vi "Main.vi"(8 "error in":errorcluster, 9 "Error Queue":refnum<queue>, 10 "Controller Queue":refnum<queue>, 11 "Application Events":refnum<user-event>) -> (0 "error out":errorcluster)   [LabVIEW 2020, in "Controller.lvlib"]
doc: "Main Vi for controller module"
uses:
  Controller.lvlib
  Controls/Module Message.ctl
  Controls/Application Modules.ctl
  Controls/Application Event Message.ctl
  Controls/Application Events.ctl
  Controls/Module Consummer Loop Data.ctl
  Controls/Module State.ctl
  Configuration Database/Configuration Database.lvlib
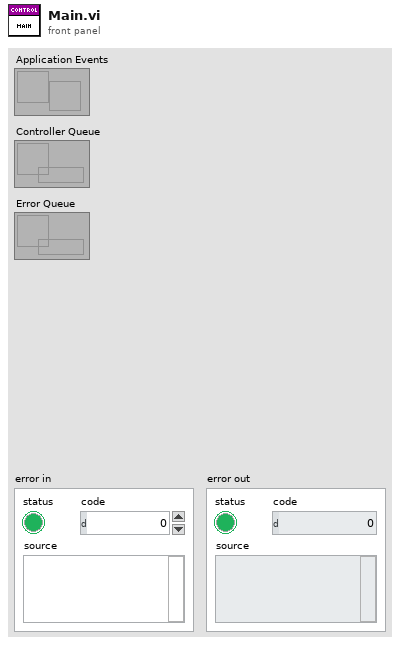
[diagram p1: front panel]
types:
  T1 = typedef "Controller.lvlib/Module State.ctl" = enum16{"Initial State", "Start And Move State", "Analysis State", "Continue Travel State", "Stop At Floor", "Open And Close Door Sequence State", "No Request Remaining State", "Emergency Call State", "Terminate Process State"}
  T2 = typedef "Controller.lvlib/Application Event Message.ctl" = cluster{"Source":T3, "Event":T4, "Data":variant}
  T3 = typedef "Controller.lvlib/Application Modules.ctl" = enum16{"Controller", "User Console", "Display Console", "Sensor Interface", "Configuration Database", "Error Module"}
  T4 = typedef "Controller.lvlib/Application Events.ctl" = enum16{"Controller: Initialize", "Controller: Initialize Start And Move State", "Controller: Initialize Analysis State", "Controller: Initialize Continue Travel State", "Controller: Initialize Stop At Floor", "Controller: Initialize Open And Close Door Sequence", "Controller: Initialize No Request Remaining", "Controller: Initialize Emergency Call", "Controller: Initialize Terminate Process", "Controller: Publish State", "UI: Elevator Call", "UI: Broadcast State", "UI: Next Destination Reached", "UI: Timeout Reached", "UI: Emergency Call", "UI: Terminate State", "UI: Door Opened", "UI: Door Closed", "UI: Floor Reached", "UI: Door About To Close"}
  T5 = typedef "Controller.lvlib/Module Consummer Loop Data.ctl" = cluster{"State Machine":cluster{"Module State":T1, "State Data":variant, "Current Operation":cluster{"Initial Floor":i32, "Elevator Calls":i32[], "Current Movement":bool}[]}}
  T6 = cluster{"Initial Floor":i32, "Elevator Calls":i32[], "Current Movement":bool}[]
  T7 = cluster{"Initial Floor":i32, "Elevator Calls":i32[], "Current Movement":bool}
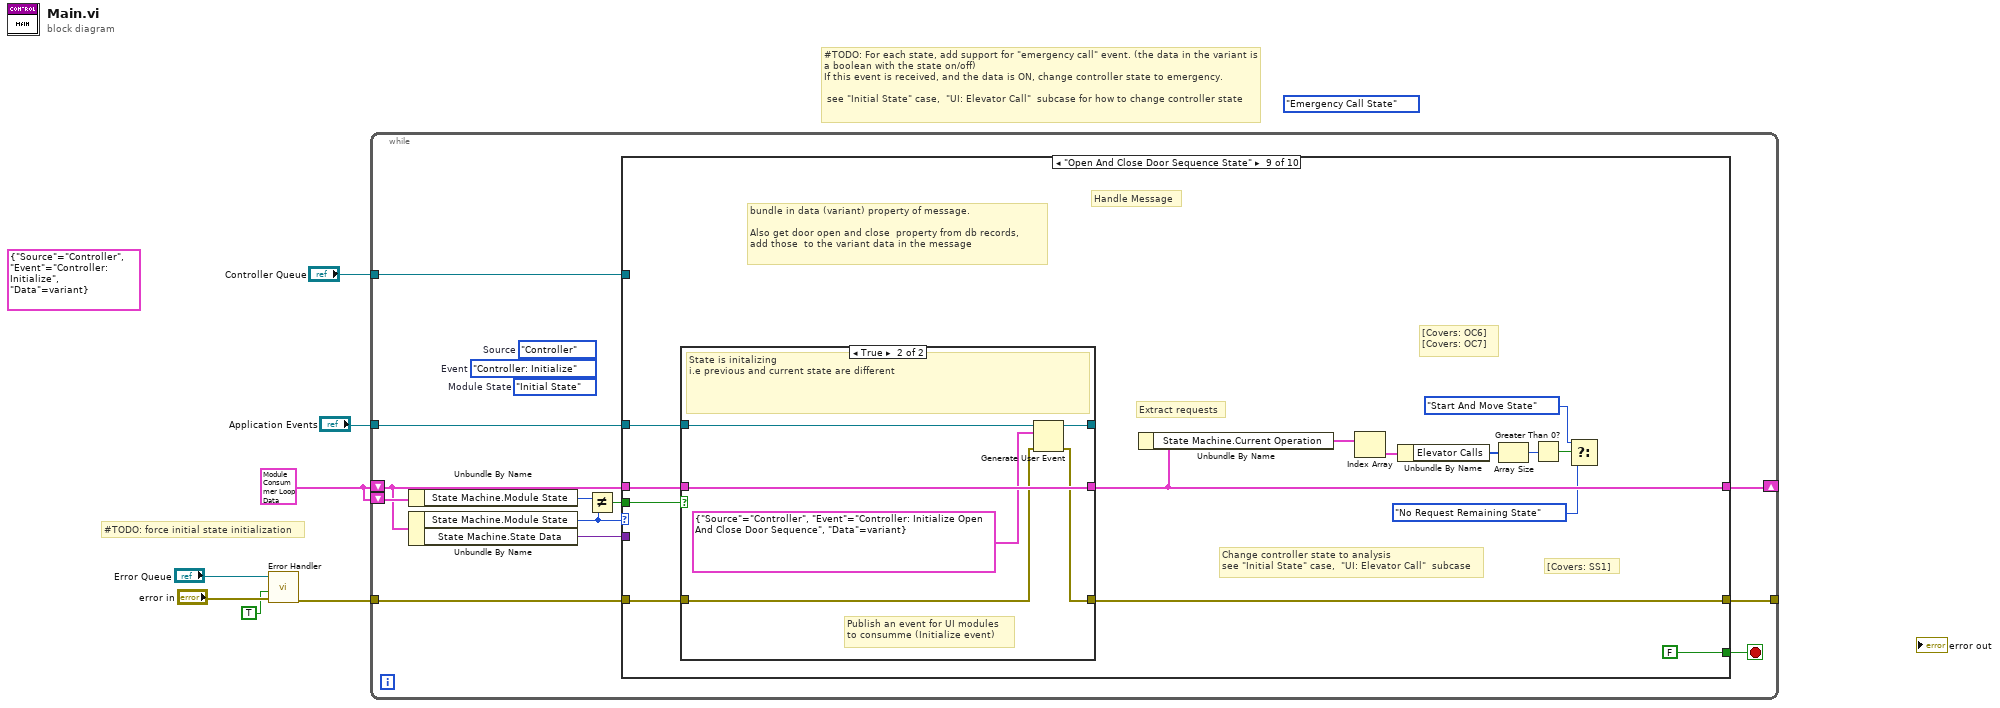
[diagram p0: block diagram]
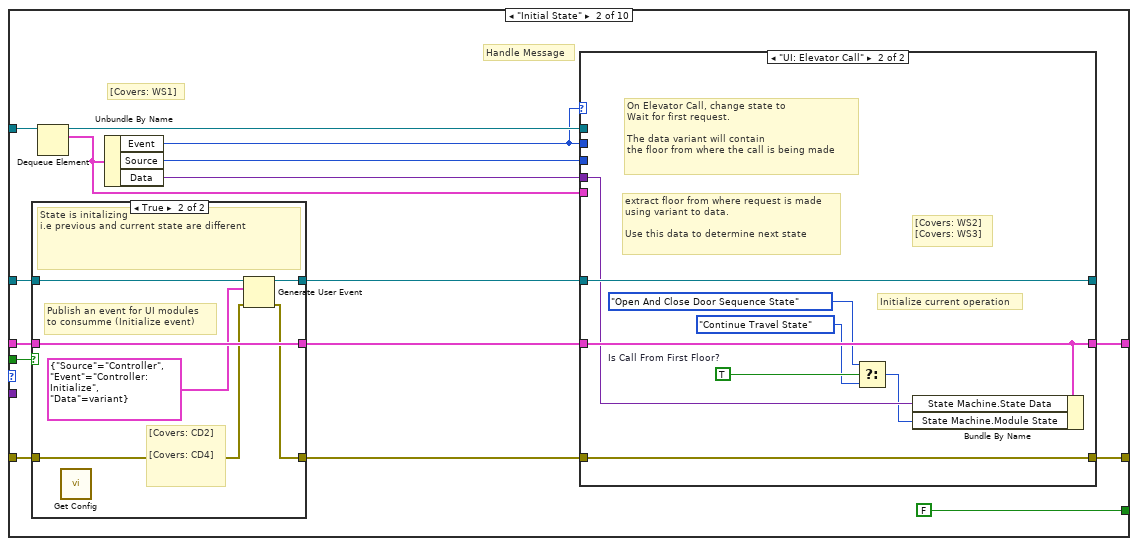
[diagram p3: hidden frame]
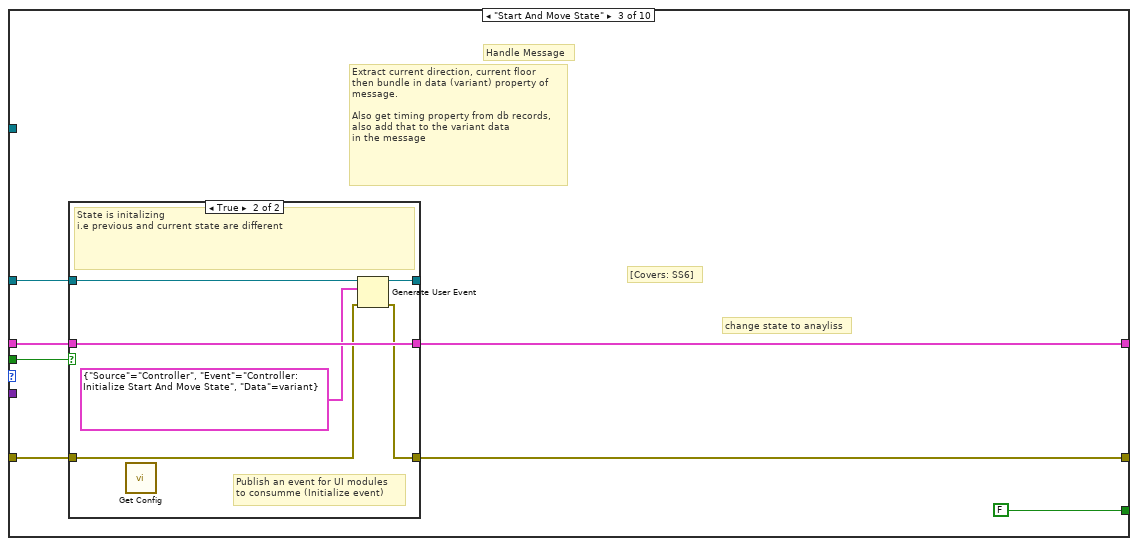
[diagram p6: hidden frame]
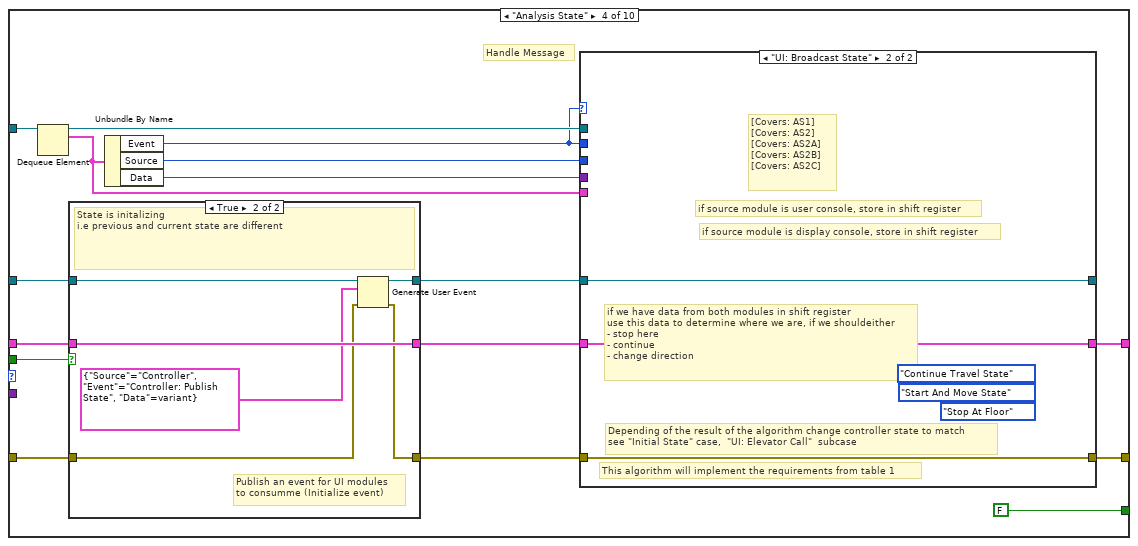
[diagram p8: hidden frame]
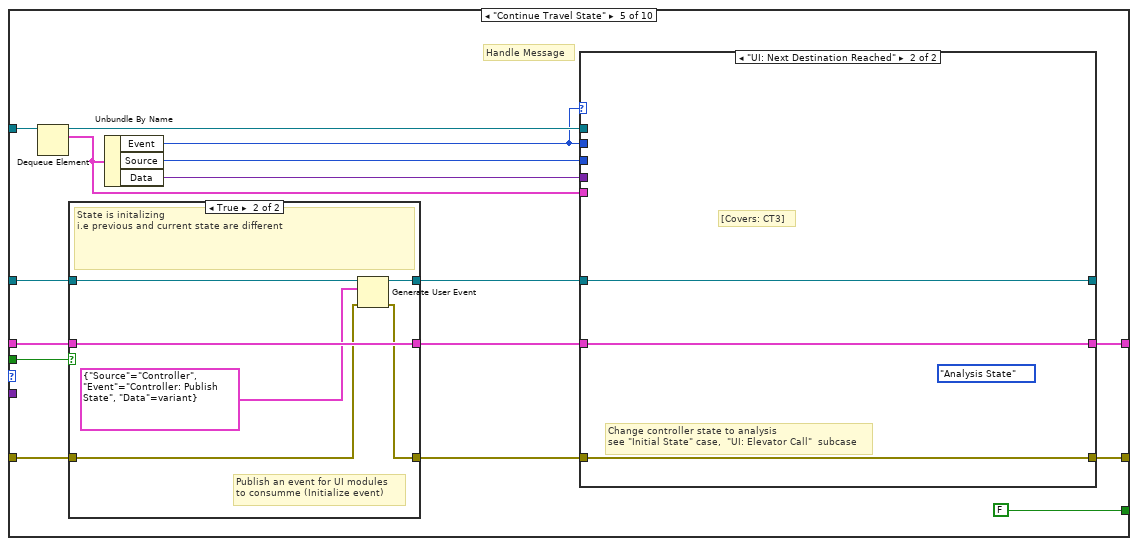
[diagram p11: hidden frame]
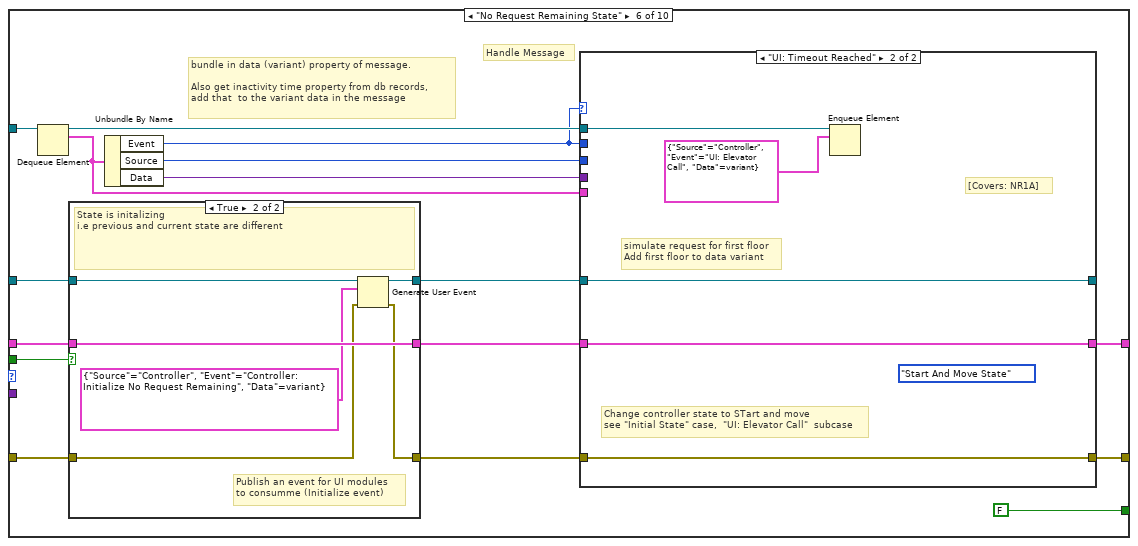
[diagram p14: hidden frame]
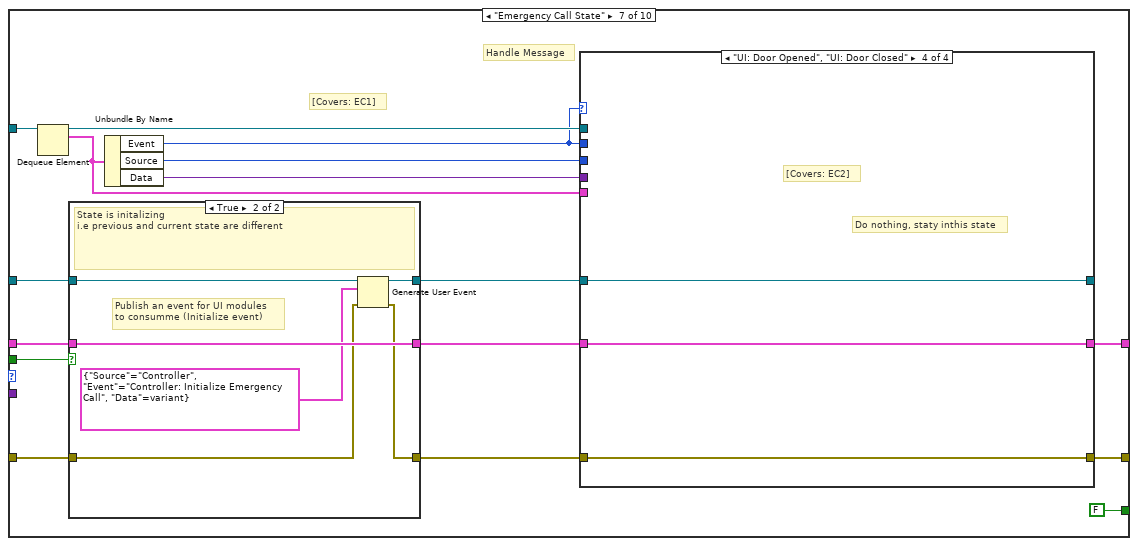
[diagram p17: hidden frame]
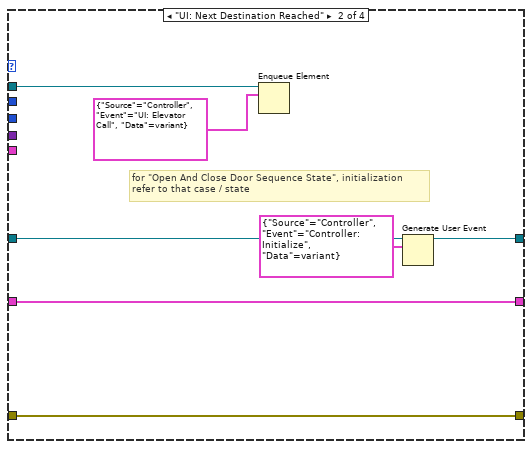
[diagram p19: hidden frame]
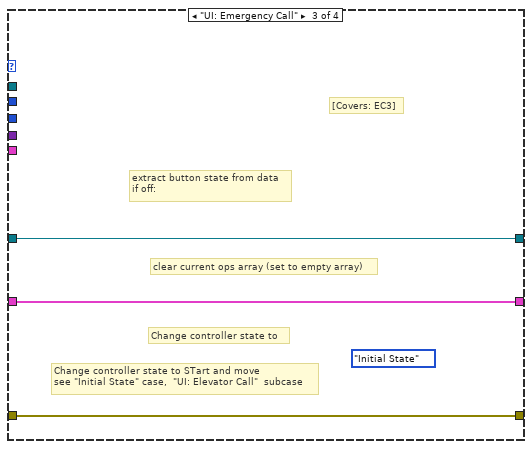
[diagram p20: hidden frame]
diagram:
  (unwired) Module_State."Emergency Call State" ("State Machine.Module State")
  (unwired) T2 {"Source"=enum."Controller", "Event"=enum."Controller: Initialize", "Data"=variant} ("Elevator Events")
  w1 = T5 {"State Machine"={"Module State"=enum."Initial State", "State Data"=variant, "Current Operation"=[]}} ("Loop Data")
  # "#TODO: For each state, add support for \"emergency call\" event. (the data in the variant is a boolean with the state on/off)\nIf this event is received, and the data is ON, change controller state to emergency.\n\n see \"Initial State\" case,  \"UI: Elevator Call\"  subcase for how to change controller state"
  # "#TODO: force initial state initialization"
  n1 = call "Error Handler.vi"("error in"="error in", "Load Reference?"=TRUE, "Error Queue"="Error Queue") -> ("error out"=w4:errorcluster)  [unwired: 8 in]
  n2 = while {
    tunnel: w4 -> [w10]
    shift-right: [w19] -> _
    shift-left: w1 -> [w17]
    shift-left: w1 -> [w18]
    tunnel: "Application Events" -> [w12]
    tunnel: "Controller Queue" -> [w11]
    tunnel: [w9] -> _
    stop <- w8 stop-if-true
    (unwired) Module_State."Initial State"  # Module State
    (unwired) Application_Events."Controller: Initialize"  # Event
    (unwired) Application_Modules."Controller"  # Source
    n3 = Unbundle By Name(w18) -> ("State Machine.Module State"=w16:T1)
    n4 = Unbundle By Name(w17) -> ("State Machine.Module State"=w15:T1, "State Machine.State Data"=w13:variant)
    n5 = Not Equal?(x=w16, y=w15) -> (x != y?=w14:bool)
    n6 = case shown="\"Open And Close Door Sequence State\"" w15 {
      tunnel: w17 -> [w21 w31 w60 w82 w112 w142 w174 w214 w239 w256]
      tunnel: [w21 w29 w58 w80 w110 w140 w172 w212 w239 w256] -> w19
      tunnel: w14 -> [_ w36 w63 w87 w117 w147 w179 w219 w244 w259]
      tunnel: w13 -> [_ _ _ _ _ _ _ _ _ _]
      tunnel: w12 -> [_ w35 w62 w86 w116 w146 w178 w218 w243 w258]
      tunnel: w11 -> [_ w34 _ w85 w115 w145 w177 w217 _ _]
      tunnel: w10 -> [w20 w33 w61 w84 w114 w144 w176 w216 w242 w257]
      tunnel: [w20 w28 w57 w79 w109 w139 w171 w211 w241 w255] -> w9
      tunnel: [_ FALSE FALSE FALSE FALSE FALSE FALSE FALSE FALSE FALSE] -> w8
      frame Default {
      }
      frame "Initial State" {
        # "[Covers: WS1]"
        # "Handle Message"
        n7 = case shown="True" w36 {
          tunnel: w31 -> [w49 w56]
          tunnel: [w49 w56] -> _
          tunnel: w35 -> [w48 w55]
          tunnel: w33 -> [w50 w52]
          tunnel: [w50 w51] -> w30
          tunnel: [w48 w54] -> w32
          frame False {
          }
          frame True {
            # "[Covers: CD2] \n\n[Covers: CD4]"
            # "Publish an event for UI modules\nto consumme (Initialize event)"
            # "State is initalizing\ni.e previous and current state are different"
            n8 = call "Get Config.vi"() -> ()  [unwired: 11 in, 1 out]
            n9 = Generate User Event(user event=w55, event data cluster=T2 {"Source"=enum."Controller", "Event"=enum."Controller: Initialize", "Data"=variant} ("event data"), error in=w52) -> (user event out=w54:refnum<user-event>, error out=w51:errorcluster)  [unwired: 1 in]
          }
        }
        n10 = Dequeue Element(queue=w34) -> (queue out=w27:refnum<queue>, element=w26:T2)  [unwired: 2 in, 2 out]
        n11 = Unbundle By Name(w26) -> ("Event"=w22:T4, "Source"=w24:T3, "Data"=w25:variant)
        n12 = case shown="\"UI: Elevator Call\"" w22 {
          tunnel: w31 -> [w38 w45]
          tunnel: [w38 w45] -> w29
          tunnel: w32 -> [w37 w46]
          tunnel: w30 -> [w39 w47]
          tunnel: [w39 w47] -> w28
          tunnel: [w37 w46] -> _
          tunnel: w27 -> [_ _]
          tunnel: w26 -> [_ _]
          tunnel: w25 -> [_ w44]
          tunnel: w24 -> [_ _]
          tunnel: w22 -> [_ _]
          frame Default {
          }
          frame "UI: Elevator Call" {
            w43 = TRUE  # Is Call From First Floor?
            # "Initialize current operation"
            # "[Covers: WS2] \n[Covers: WS3]"
            # "extract floor from where request is made\nusing variant to data.\n\nUse this data to determine next state"
            # "On Elevator Call, change state to\nWait for first request.\n\nThe data variant will contain\nthe floor from where the call is being made"
            n13 = Select(t=Module_State."Open And Close Door Sequence State" ("State Machine.Module State"), s=w43, f=Module_State."Continue Travel State" ("State Machine.Module State")) -> (s? t:f=w42:T1)
            n14 = Bundle By Name(cluster=w45, "State Machine.State Data"=w44, "State Machine.Module State"=w42) -> ()  [unwired: 1 out]
          }
        }
      }
      frame "Start And Move State" {
        # "change state to anayliss"
        # "[Covers: SS6]"
        # "Extract current direction, current floor\nthen bundle in data (variant) property of message.\n\nAlso get timing property from db records, also add that to the variant data\nin the message"
        # "Handle Message"
        n15 = case shown="True" w63 {
          tunnel: w60 -> [w65 w72]
          tunnel: [w65 w72] -> w58
          tunnel: w62 -> [w64 w71]
          tunnel: w61 -> [w66 w68]
          tunnel: [w66 w67] -> w57
          tunnel: [w64 w70] -> _
          frame False {
          }
          frame True {
            # "Publish an event for UI modules\nto consumme (Initialize event)"
            # "State is initalizing\ni.e previous and current state are different"
            n16 = call "Get Config.vi"() -> ()  [unwired: 11 in, 1 out]
            n17 = Generate User Event(user event=w71, event data cluster=T2 {"Source"=enum."Controller", "Event"=enum."Controller: Initialize Start And Move State", "Data"=variant} ("event data"), error in=w68) -> (user event out=w70:refnum<user-event>, error out=w67:errorcluster)  [unwired: 1 in]
          }
        }
      }
      frame "Analysis State" {
        # "Handle Message"
        n18 = Dequeue Element(queue=w85) -> (queue out=w78:refnum<queue>, element=w77:T2)  [unwired: 2 in, 2 out]
        n19 = case shown="True" w87 {
          tunnel: w82 -> [w95 w102]
          tunnel: [w95 w102] -> _
          tunnel: w86 -> [w94 w101]
          tunnel: w84 -> [w96 w98]
          tunnel: [w96 w97] -> w81
          tunnel: [w94 w100] -> w83
          frame False {
          }
          frame True {
            # "Publish an event for UI modules\nto consumme (Initialize event)"
            # "State is initalizing\ni.e previous and current state are different"
            n20 = Generate User Event(user event=w101, event data cluster=T2 {"Source"=enum."Controller", "Event"=enum."Controller: Publish State", "Data"=variant} ("event data"), error in=w98) -> (user event out=w100:refnum<user-event>, error out=w97:errorcluster)  [unwired: 1 in]
          }
        }
        n21 = Unbundle By Name(w77) -> ("Event"=w73:T4, "Source"=w75:T3, "Data"=w76:variant)
        n22 = case shown="\"UI: Broadcast State\"" w73 {
          tunnel: w82 -> [w89 w93]
          tunnel: [w89 w93] -> w80
          tunnel: w83 -> [w88 w91]
          tunnel: w81 -> [w90 w92]
          tunnel: [w90 w92] -> w79
          tunnel: [w88 w91] -> _
          tunnel: w78 -> [_ _]
          tunnel: w77 -> [_ _]
          tunnel: w76 -> [_ _]
          tunnel: w75 -> [_ _]
          tunnel: w73 -> [_ _]
          frame Default {
          }
          frame "UI: Broadcast State" {
            (unwired) Module_State."Stop At Floor" ("State Machine.Module State")
            (unwired) Module_State."Start And Move State" ("State Machine.Module State")
            (unwired) Module_State."Continue Travel State" ("State Machine.Module State")
            # "[Covers: AS1] \n[Covers: AS2] \n[Covers: AS2A] \n[Covers: AS2B] \n[Covers: AS2C]"
            # "Depending of the result of the algorithm change controller state to match\nsee \"Initial State\" case,  \"UI: Elevator Call\"  subcase"
            # "This algorithm will implement the requirements from table 1"
            # "if we have data from both modules in shift register\nuse this data to determine where we are, if we shouldeither\n- stop here\n- continue\n- change direction"
            # "if source module is display console, store in shift register"
            # "if source module is user console, store in shift register"
          }
        }
      }
      frame "Continue Travel State" {
        # "Handle Message"
        n23 = Dequeue Element(queue=w115) -> (queue out=w108:refnum<queue>, element=w107:T2)  [unwired: 2 in, 2 out]
        n24 = case shown="True" w117 {
          tunnel: w112 -> [w125 w132]
          tunnel: [w125 w132] -> _
          tunnel: w116 -> [w124 w131]
          tunnel: w114 -> [w126 w128]
          tunnel: [w126 w127] -> w111
          tunnel: [w124 w130] -> w113
          frame False {
          }
          frame True {
            # "Publish an event for UI modules\nto consumme (Initialize event)"
            # "State is initalizing\ni.e previous and current state are different"
            n25 = Generate User Event(user event=w131, event data cluster=T2 {"Source"=enum."Controller", "Event"=enum."Controller: Publish State", "Data"=variant} ("event data"), error in=w128) -> (user event out=w130:refnum<user-event>, error out=w127:errorcluster)  [unwired: 1 in]
          }
        }
        n26 = Unbundle By Name(w107) -> ("Event"=w103:T4, "Source"=w105:T3, "Data"=w106:variant)
        n27 = case shown="\"UI: Next Destination Reached\"" w103 {
          tunnel: w112 -> [w119 w123]
          tunnel: [w119 w123] -> w110
          tunnel: w113 -> [w118 w121]
          tunnel: w111 -> [w120 w122]
          tunnel: [w120 w122] -> w109
          tunnel: [w118 w121] -> _
          tunnel: w108 -> [_ _]
          tunnel: w107 -> [_ _]
          tunnel: w106 -> [_ _]
          tunnel: w105 -> [_ _]
          tunnel: w103 -> [_ _]
          frame Default {
          }
          frame "UI: Next Destination Reached" {
            (unwired) Module_State."Analysis State" ("State Machine.Module State")
            # "[Covers: CT3]"
            # "Change controller state to analysis\nsee \"Initial State\" case,  \"UI: Elevator Call\"  subcase"
          }
        }
      }
      frame "No Request Remaining State" {
        # "bundle in data (variant) property of message.\n\nAlso get inactivity time property from db records, \nadd that  to the variant data in the message"
        # "Handle Message"
        n28 = Dequeue Element(queue=w145) -> (queue out=w138:refnum<queue>, element=w137:T2)  [unwired: 2 in, 2 out]
        n29 = case shown="True" w147 {
          tunnel: w142 -> [w157 w164]
          tunnel: [w157 w164] -> _
          tunnel: w146 -> [w156 w163]
          tunnel: w144 -> [w158 w160]
          tunnel: [w158 w159] -> w141
          tunnel: [w156 w162] -> w143
          frame False {
          }
          frame True {
            # "Publish an event for UI modules\nto consumme (Initialize event)"
            # "State is initalizing\ni.e previous and current state are different"
            n30 = Generate User Event(user event=w163, event data cluster=T2 {"Source"=enum."Controller", "Event"=enum."Controller: Initialize No Request Remaining", "Data"=variant} ("event data"), error in=w160) -> (user event out=w162:refnum<user-event>, error out=w159:errorcluster)  [unwired: 1 in]
          }
        }
        n31 = Unbundle By Name(w137) -> ("Event"=w133:T4, "Source"=w135:T3, "Data"=w136:variant)
        n32 = case shown="\"UI: Timeout Reached\"" w133 {
          tunnel: w142 -> [w149 w155]
          tunnel: [w149 w155] -> w140
          tunnel: w143 -> [w148 w153]
          tunnel: w141 -> [w150 w154]
          tunnel: [w150 w154] -> w139
          tunnel: [w148 w153] -> _
          tunnel: w138 -> [_ w152]
          tunnel: w137 -> [_ _]
          tunnel: w136 -> [_ _]
          tunnel: w135 -> [_ _]
          tunnel: w133 -> [_ _]
          frame Default {
          }
          frame "UI: Timeout Reached" {
            (unwired) Module_State."Start And Move State" ("State Machine.Module State")
            # "[Covers: NR1A]"
            # "simulate request for first floor\nAdd first floor to data variant"
            # "Change controller state to STart and move\nsee \"Initial State\" case,  \"UI: Elevator Call\"  subcase"
            n33 = Enqueue Element(queue=w152, element=T2 {"Source"=enum."Controller", "Event"=enum."UI: Elevator Call", "Data"=variant}) -> ()  [unwired: 2 in, 3 out]
          }
        }
      }
      frame "Emergency Call State" {
        # "[Covers: EC1]"
        # "Handle Message"
        n34 = Dequeue Element(queue=w177) -> (queue out=w170:refnum<queue>, element=w169:T2)  [unwired: 2 in, 2 out]
        n35 = case shown="True" w179 {
          tunnel: w174 -> [w197 w204]
          tunnel: [w197 w204] -> _
          tunnel: w178 -> [w196 w203]
          tunnel: w176 -> [w198 w200]
          tunnel: [w198 w199] -> w173
          tunnel: [w196 w202] -> w175
          frame False {
          }
          frame True {
            # "Publish an event for UI modules\nto consumme (Initialize event)"
            # "State is initalizing\ni.e previous and current state are different"
            n36 = Generate User Event(user event=w203, event data cluster=T2 {"Source"=enum."Controller", "Event"=enum."Controller: Initialize Emergency Call", "Data"=variant} ("event data"), error in=w200) -> (user event out=w202:refnum<user-event>, error out=w199:errorcluster)  [unwired: 1 in]
          }
        }
        n37 = Unbundle By Name(w169) -> ("Event"=w165:T4, "Source"=w167:T3, "Data"=w168:variant)
        n38 = case shown="\"UI: Door Opened\", \"UI: Door Closed\"" w165 {
          tunnel: w174 -> [w181 w189 w192 w195]
          tunnel: [w181 w189 w192 w195] -> w172
          tunnel: w175 -> [w180 w185 w190 w193]
          tunnel: w173 -> [w182 w188 w191 w194]
          tunnel: [w182 w188 w191 w194] -> w171
          tunnel: [w180 w184 w190 w193] -> _
          tunnel: w170 -> [_ w187 _ _]
          tunnel: w169 -> [_ _ _ _]
          tunnel: w168 -> [_ _ _ _]
          tunnel: w167 -> [_ _ _ _]
          tunnel: w165 -> [_ _ _ _]
          frame Default {
          }
          frame "UI: Next Destination Reached" {
            # "for \"Open And Close Door Sequence State\", initialization\nrefer to that case / state"
            n39 = Enqueue Element(queue=w187, element=T2 {"Source"=enum."Controller", "Event"=enum."UI: Elevator Call", "Data"=variant}) -> ()  [unwired: 2 in, 3 out]
            n40 = Generate User Event(user event=w185, event data cluster=T2 {"Source"=enum."Controller", "Event"=enum."Controller: Initialize", "Data"=variant} ("event data")) -> (user event out=w184:refnum<user-event>)  [unwired: 2 in, 1 out]
          }
          frame "UI: Emergency Call" {
            (unwired) Module_State."Initial State" ("State Machine.Module State")
            # "[Covers: EC3]"
            # "Change controller state to STart and move\nsee \"Initial State\" case,  \"UI: Elevator Call\"  subcase"
            # "Change controller state to"
            # "clear current ops array (set to empty array)"
            # "extract button state from data\nif off:"
          }
          frame "UI: Door Opened", "UI: Door Closed" {
            # "Do nothing, staty inthis state"
            # "[Covers: EC2]"
          }
        }
      }
      frame "Terminate Process State" {
        # "Handle Message"
        n41 = Dequeue Element(queue=w217) -> (queue out=w210:refnum<queue>, element=w209:T2)  [unwired: 2 in, 2 out]
        n42 = case shown="True" w219 {
          tunnel: w214 -> [w224 w231]
          tunnel: [w224 w231] -> _
          tunnel: w218 -> [w223 w230]
          tunnel: w216 -> [w225 w227]
          tunnel: [w225 w226] -> w213
          tunnel: [w223 w229] -> w215
          frame False {
          }
          frame True {
            # "Publish an event for UI modules\nto consumme (Initialize event)"
            # "State is initalizing\ni.e previous and current state are different"
            n43 = Generate User Event(user event=w230, event data cluster=T2 {"Source"=enum."Controller", "Event"=enum."Controller: Initialize Terminate Process", "Data"=variant} ("event data"), error in=w227) -> (user event out=w229:refnum<user-event>, error out=w226:errorcluster)  [unwired: 1 in]
          }
        }
        n44 = Unbundle By Name(w209) -> ("Event"=w205:T4, "Source"=w207:T3, "Data"=w208:variant)
        n45 = case shown="Default" w205 {
          tunnel: w214 -> [w221]
          tunnel: [w221] -> w212
          tunnel: w215 -> [w220]
          tunnel: w213 -> [w222]
          tunnel: [w222] -> w211
          tunnel: [w220] -> _
          tunnel: w210 -> [_]
          tunnel: w209 -> [_]
          tunnel: w208 -> [_]
          tunnel: w207 -> [_]
          tunnel: w205 -> [_]
          frame Default {
          }
        }
      }
      frame "Open And Close Door Sequence State" {
        # "[Covers: SS1]"
        # "[Covers: OC6]\n[Covers: OC7]"
        # "Extract requests"
        # "Change controller state to analysis\nsee \"Initial State\" case,  \"UI: Elevator Call\"  subcase"
        # "bundle in data (variant) property of message.\n\nAlso get door open and close  property from db records, \nadd those  to the variant data in the message"
        # "Handle Message"
        n46 = case shown="True" w244 {
          tunnel: w239 -> [w246 w253]
          tunnel: [w246 w253] -> _
          tunnel: w243 -> [w245 w252]
          tunnel: w242 -> [w247 w249]
          tunnel: [w247 w248] -> w241
          tunnel: [w245 w251] -> _
          frame False {
          }
          frame True {
            # "Publish an event for UI modules\nto consumme (Initialize event)"
            # "State is initalizing\ni.e previous and current state are different"
            n47 = Generate User Event(user event=w252, event data cluster=T2 {"Source"=enum."Controller", "Event"=enum."Controller: Initialize Open And Close Door Sequence", "Data"=variant} ("event data"), error in=w249) -> (user event out=w251:refnum<user-event>, error out=w248:errorcluster)  [unwired: 1 in]
          }
        }
        n48 = Unbundle By Name(w239) -> ("State Machine.Current Operation"=w238:T6)
        n49 = Index Array(array=w238) -> (element=w237:T7)  [unwired: 1 in]
        n50 = Unbundle By Name(w237) -> ("Elevator Calls"=w236:i32[])
        n51 = Array Size(array=w236) -> (size(s)=w235:i32)
        n52 = Greater Than 0?(x=w235) -> (x > 0?=w234:bool)
        n53 = Select(t=Module_State."Start And Move State" ("State Machine.Module State"), s=w234, f=Module_State."No Request Remaining State" ("State Machine.Module State")) -> ()  [unwired: 1 out]
      }
      frame "Stop At Floor" {
        (unwired) Module_State."Open And Close Door Sequence State" ("State Machine.Module State")
        # "[Covers: RF3]"
        # "Change controller state to Open and Close Door Sequence\nsee \"Initial State\" case,  \"UI: Elevator Call\"  subcase"
        n54 = case shown="True" w259 {
          tunnel: w256 -> [w261 w268]
          tunnel: [w261 w268] -> _
          tunnel: w258 -> [w260 w267]
          tunnel: w257 -> [w262 w264]
          tunnel: [w262 w263] -> w255
          tunnel: [w260 w266] -> _
          frame False {
          }
          frame True {
            # "Publish an event for UI modules\nto consumme (Initialize event)"
            # "State is initalizing\ni.e previous and current state are different"
            n55 = Generate User Event(user event=w267, event data cluster=T2 {"Source"=enum."Controller", "Event"=enum."Controller: Initialize Stop At Floor", "Data"=variant} ("event data"), error in=w264) -> (user event out=w266:refnum<user-event>, error out=w263:errorcluster)  [unwired: 1 in]
          }
        }
      }
    }
  }
